vi "DDS_Clock.vi"() -> ()   [LabVIEW 2016] (continued)
"f1 [Hz] CH0"=307800000.0}, {"total time[ms]"=68.04999999999828, "f1 [Hz] CH0"=307800000.0}, {"total time[ms]"=68.09999999999827, "f1 [Hz] CH0"=307599999.99999994}, {"total time[ms]"=68.09999999999827, "f1 [Hz] CH0"=307599999.99999994}, {"total time[ms]"=68.14999999999827, "f1 [Hz] CH0"=307399999.99999994}, {"total time[ms]"=68.14999999999827, "f1 [Hz] CH0"=307399999.99999994}, {"total time[ms]"=68.19999999999827, "f1 [Hz] CH0"=307200000.0}, {"total time[ms]"=68.19999999999827, "f1 [Hz] CH0"=307200000.0}, {"total time[ms]"=68.24999999999827, "f1 [Hz] CH0"=307000000.0}, {"total time[ms]"=68.24999999999827, "f1 [Hz] CH0"=307000000.0}, {"total time[ms]"=68.29999999999826, "f1 [Hz] CH0"=306800000.0}, {"total time[ms]"=68.29999999999826, "f1 [Hz] CH0"=306800000.0}, {"total time[ms]"=68.34999999999826, "f1 [Hz] CH0"=306599999.99999994}, {"total time[ms]"=68.34999999999826, "f1 [Hz] CH0"=306599999.99999994}, {"total time[ms]"=68.39999999999826, "f1 [Hz] CH0"=306400000.0}, {"total time[ms]"=68.39999999999826, "f1 [Hz] CH0"=306400000.0}, {"total time[ms]"=68.44999999999825, "f1 [Hz] CH0"=306200000.0}, {"total time[ms]"=68.44999999999825, "f1 [Hz] CH0"=306200000.0}, {"total time[ms]"=68.49999999999825, "f1 [Hz] CH0"=306000000.0}, {"total time[ms]"=68.49999999999825, "f1 [Hz] CH0"=306000000.0}, {"total time[ms]"=68.54999999999825, "f1 [Hz] CH0"=305800000.0}, {"total time[ms]"=68.54999999999825, "f1 [Hz] CH0"=305800000.0}, {"total time[ms]"=68.59999999999825, "f1 [Hz] CH0"=305599999.99999994}, {"total time[ms]"=68.59999999999825, "f1 [Hz] CH0"=305599999.99999994}, {"total time[ms]"=68.64999999999824, "f1 [Hz] CH0"=305399999.99999994}, {"total time[ms]"=68.64999999999824, "f1 [Hz] CH0"=305399999.99999994}, {"total time[ms]"=68.69999999999824, "f1 [Hz] CH0"=305199999.99999994}, {"total time[ms]"=68.69999999999824, "f1 [Hz] CH0"=305199999.99999994}, {"total time[ms]"=68.74999999999824, "f1 [Hz] CH0"=305000000.0}, {"total time[ms]"=68.74999999999824, "f1 [Hz] CH0"=305000000.0}, {"total time[ms]"=68.79999999999824, "f1 [Hz] CH0"=304800000.0}, {"total time[ms]"=68.79999999999824, "f1 [Hz] CH0"=304800000.0}, {"total time[ms]"=68.84999999999823, "f1 [Hz] CH0"=304599999.99999994}, {"total time[ms]"=68.84999999999823, "f1 [Hz] CH0"=304599999.99999994}, {"total time[ms]"=68.89999999999823, "f1 [Hz] CH0"=304400000.0}, {"total time[ms]"=68.89999999999823, "f1 [Hz] CH0"=304400000.0}, {"total time[ms]"=68.94999999999823, "f1 [Hz] CH0"=304200000.0}, {"total time[ms]"=68.94999999999823, "f1 [Hz] CH0"=304200000.0}, {"total time[ms]"=68.99999999999822, "f1 [Hz] CH0"=304000000.0}, {"total time[ms]"=68.99999999999822, "f1 [Hz] CH0"=304000000.0}, {"total time[ms]"=69.04999999999822, "f1 [Hz] CH0"=303800000.0}, {"total time[ms]"=69.04999999999822, "f1 [Hz] CH0"=303800000.0}, {"total time[ms]"=69.09999999999822, "f1 [Hz] CH0"=303599999.99999994}, {"total time[ms]"=69.09999999999822, "f1 [Hz] CH0"=303599999.99999994}, {"total time[ms]"=69.14999999999822, "f1 [Hz] CH0"=303399999.99999994}, {"total time[ms]"=69.14999999999822, "f1 [Hz] CH0"=303399999.99999994}, {"total time[ms]"=69.19999999999821, "f1 [Hz] CH0"=303199999.99999994}, {"total time[ms]"=69.19999999999821, "f1 [Hz] CH0"=303199999.99999994}, {"total time[ms]"=69.24999999999821, "f1 [Hz] CH0"=303000000.0}, {"total time[ms]"=69.24999999999821, "f1 [Hz] CH0"=303000000.0}, {"total time[ms]"=69.2999999999982, "f1 [Hz] CH0"=302800000.0}, {"total time[ms]"=69.2999999999982, "f1 [Hz] CH0"=302800000.0}, {"total time[ms]"=69.3499999999982, "f1 [Hz] CH0"=302599999.99999994}, {"total time[ms]"=69.3499999999982, "f1 [Hz] CH0"=302599999.99999994}, {"total time[ms]"=69.3999999999982, "f1 [Hz] CH0"=302399999.99999994}, {"total time[ms]"=69.3999999999982, "f1 [Hz] CH0"=302399999.99999994}, {"total time[ms]"=69.4499999999982, "f1 [Hz] CH0"=302200000.0}, {"total time[ms]"=69.4499999999982, "f1 [Hz] CH0"=302200000.0}, {"total time[ms]"=69.4999999999982, "f1 [Hz] CH0"=302000000.0}, {"total time[ms]"=69.4999999999982, "f1 [Hz] CH0"=302000000.0}, {"total time[ms]"=69.54999999999819, "f1 [Hz] CH0"=301800000.0}, {"total time[ms]"=69.54999999999819, "f1 [Hz] CH0"=301800000.0}, {"total time[ms]"=69.59999999999819, "f1 [Hz] CH0"=301599999.99999994}, {"total time[ms]"=69.59999999999819, "f1 [Hz] CH0"=301599999.99999994}, {"total time[ms]"=69.64999999999819, "f1 [Hz] CH0"=301400000.0}, {"total time[ms]"=69.64999999999819, "f1 [Hz] CH0"=301400000.0}, {"total time[ms]"=69.69999999999818, "f1 [Hz] CH0"=301200000.0}, {"total time[ms]"=69.69999999999818, "f1 [Hz] CH0"=301200000.0}, {"total time[ms]"=69.74999999999818, "f1 [Hz] CH0"=301000000.0}, {"total time[ms]"=69.74999999999818, "f1 [Hz] CH0"=301000000.0}, {"total time[ms]"=69.79999999999818, "f1 [Hz] CH0"=300800000.0}, {"total time[ms]"=69.79999999999818, "f1 [Hz] CH0"=300800000.0}, {"total time[ms]"=69.84999999999818, "f1 [Hz] CH0"=300599999.99999994}, {"total time[ms]"=69.84999999999818, "f1 [Hz] CH0"=300599999.99999994}, {"total time[ms]"=69.89999999999817, "f1 [Hz] CH0"=300399999.99999994}, {"total time[ms]"=69.89999999999817, "f1 [Hz] CH0"=300399999.99999994}, {"total time[ms]"=69.94999999999817, "f1 [Hz] CH0"=300199999.99999994}, {"total time[ms]"=69.94999999999817, "f1 [Hz] CH0"=300199999.99999994}, {"total time[ms]"=69.99999999999817, "f1 [Hz] CH0"=300000000.0}, {"total time[ms]"=69.99999999999817, "f1 [Hz] CH0"=300000000.0}, {"total time[ms]"=70.04999999999816, "f1 [Hz] CH0"=300200000.0}, {"total time[ms]"=70.04999999999816, "f1 [Hz] CH0"=300200000.0}, {"total time[ms]"=70.09999999999816, "f1 [Hz] CH0"=300400000.00000006}, {"total time[ms]"=70.09999999999816, "f1 [Hz] CH0"=300400000.00000006}, {"total time[ms]"=70.14999999999816, "f1 [Hz] CH0"=300600000.0}, {"total time[ms]"=70.14999999999816, "f1 [Hz] CH0"=300600000.0}, {"total time[ms]"=70.19999999999816, "f1 [Hz] CH0"=300800000.0}, {"total time[ms]"=70.19999999999816, "f1 [Hz] CH0"=300800000.0}, {"total time[ms]"=70.24999999999815, "f1 [Hz] CH0"=301000000.0}, {"total time[ms]"=70.24999999999815, "f1 [Hz] CH0"=301000000.0}, {"total time[ms]"=70.29999999999815, "f1 [Hz] CH0"=301200000.0}, {"total time[ms]"=70.29999999999815, "f1 [Hz] CH0"=301200000.0}, {"total time[ms]"=70.34999999999815, "f1 [Hz] CH0"=301400000.00000006}, {"total time[ms]"=70.34999999999815, "f1 [Hz] CH0"=301400000.00000006}, {"total time[ms]"=70.39999999999814, "f1 [Hz] CH0"=301600000.00000006}, {"total time[ms]"=70.39999999999814, "f1 [Hz] CH0"=301600000.00000006}, {"total time[ms]"=70.44999999999814, "f1 [Hz] CH0"=301800000.00000006}, {"total time[ms]"=70.44999999999814, "f1 [Hz] CH0"=301800000.00000006}, {"total time[ms]"=70.49999999999814, "f1 [Hz] CH0"=302000000.0}, {"total time[ms]"=70.49999999999814, "f1 [Hz] CH0"=302000000.0}, {"total time[ms]"=70.54999999999814, "f1 [Hz] CH0"=302200000.0}, {"total time[ms]"=70.54999999999814, "f1 [Hz] CH0"=302200000.0}, {"total time[ms]"=70.59999999999813, "f1 [Hz] CH0"=302400000.00000006}, {"total time[ms]"=70.59999999999813, "f1 [Hz] CH0"=302400000.00000006}, {"total time[ms]"=70.64999999999813, "f1 [Hz] CH0"=302600000.00000006}, {"total time[ms]"=70.64999999999813, "f1 [Hz] CH0"=302600000.00000006}, {"total time[ms]"=70.69999999999813, "f1 [Hz] CH0"=302800000.0}, {"total time[ms]"=70.69999999999813, "f1 [Hz] CH0"=302800000.0}, {"total time[ms]"=70.74999999999812, "f1 [Hz] CH0"=303000000.0}, {"total time[ms]"=70.74999999999812, "f1 [Hz] CH0"=303000000.0}, {"total time[ms]"=70.79999999999812, "f1 [Hz] CH0"=303200000.0}, {"total time[ms]"=70.79999999999812, "f1 [Hz] CH0"=303200000.0}, {"total time[ms]"=70.84999999999812, "f1 [Hz] CH0"=303400000.00000006}, {"total time[ms]"=70.84999999999812, "f1 [Hz] CH0"=303400000.00000006}, {"total time[ms]"=70.89999999999812, "f1 [Hz] CH0"=303600000.0}, {"total time[ms]"=70.89999999999812, "f1 [Hz] CH0"=303600000.0}, {"total time[ms]"=70.94999999999811, "f1 [Hz] CH0"=303800000.0}, {"total time[ms]"=70.94999999999811, "f1 [Hz] CH0"=303800000.0}, {"total time[ms]"=70.99999999999811, "f1 [Hz] CH0"=304000000.0}, {"total time[ms]"=70.99999999999811, "f1 [Hz] CH0"=304000000.0}, {"total time[ms]"=71.04999999999811, "f1 [Hz] CH0"=304200000.0}, {"total time[ms]"=71.04999999999811, "f1 [Hz] CH0"=304200000.0}, {"total time[ms]"=71.0999999999981, "f1 [Hz] CH0"=304400000.00000006}, {"total time[ms]"=71.0999999999981, "f1 [Hz] CH0"=304400000.00000006}, {"total time[ms]"=71.1499999999981, "f1 [Hz] CH0"=304600000.00000006}, {"total time[ms]"=71.1499999999981, "f1 [Hz] CH0"=304600000.00000006}, {"total time[ms]"=71.1999999999981, "f1 [Hz] CH0"=304800000.00000006}, {"total time[ms]"=71.1999999999981, "f1 [Hz] CH0"=304800000.00000006}, {"total time[ms]"=71.2499999999981, "f1 [Hz] CH0"=305000000.0}, {"total time[ms]"=71.2499999999981, "f1 [Hz] CH0"=305000000.0}, {"total time[ms]"=71.2999999999981, "f1 [Hz] CH0"=305200000.0}, {"total time[ms]"=71.2999999999981, "f1 [Hz] CH0"=305200000.0}, {"total time[ms]"=71.34999999999809, "f1 [Hz] CH0"=305400000.00000006}, {"total time[ms]"=71.34999999999809, "f1 [Hz] CH0"=305400000.00000006}, {"total time[ms]"=71.39999999999809, "f1 [Hz] CH0"=305600000.0}, {"total time[ms]"=71.39999999999809, "f1 [Hz] CH0"=305600000.0}, {"total time[ms]"=71.44999999999808, "f1 [Hz] CH0"=305800000.0}, {"total time[ms]"=71.44999999999808, "f1 [Hz] CH0"=305800000.0}, {"total time[ms]"=71.49999999999808, "f1 [Hz] CH0"=306000000.0}, {"total time[ms]"=71.49999999999808, "f1 [Hz] CH0"=306000000.0}, {"total time[ms]"=71.54999999999808, "f1 [Hz] CH0"=306200000.0}, {"total time[ms]"=71.54999999999808, "f1 [Hz] CH0"=306200000.0}, {"total time[ms]"=71.59999999999808, "f1 [Hz] CH0"=306400000.00000006}, {"total time[ms]"=71.59999999999808, "f1 [Hz] CH0"=306400000.00000006}, {"total time[ms]"=71.64999999999807, "f1 [Hz] CH0"=306600000.00000006}, {"total time[ms]"=71.64999999999807, "f1 [Hz] CH0"=306600000.00000006}, {"total time[ms]"=71.69999999999807, "f1 [Hz] CH0"=306800000.00000006}, {"total time[ms]"=71.69999999999807, "f1 [Hz] CH0"=306800000.00000006}, {"total time[ms]"=71.74999999999807, "f1 [Hz] CH0"=307000000.0}, {"total time[ms]"=71.74999999999807, "f1 [Hz] CH0"=307000000.0}, {"total time[ms]"=71.79999999999806, "f1 [Hz] CH0"=307200000.0}, {"total time[ms]"=71.79999999999806, "f1 [Hz] CH0"=307200000.0}, {"total time[ms]"=71.84999999999806, "f1 [Hz] CH0"=307400000.00000006}, {"total time[ms]"=71.84999999999806, "f1 [Hz] CH0"=307400000.00000006}, {"total time[ms]"=71.89999999999806, "f1 [Hz] CH0"=307600000.00000006}, {"total time[ms]"=71.89999999999806, "f1 [Hz] CH0"=307600000.00000006}, {"total time[ms]"=71.94999999999806, "f1 [Hz] CH0"=307800000.0}, {"total time[ms]"=71.94999999999806, "f1 [Hz] CH0"=307800000.0}, {"total time[ms]"=71.99999999999805, "f1 [Hz] CH0"=308000000.0}, {"total time[ms]"=71.99999999999805, "f1 [Hz] CH0"=308000000.0}, {"total time[ms]"=72.04999999999805, "f1 [Hz] CH0"=308200000.0}, {"total time[ms]"=72.04999999999805, "f1 [Hz] CH0"=308200000.0}, {"total time[ms]"=72.09999999999805, "f1 [Hz] CH0"=308400000.00000006}, {"total time[ms]"=72.09999999999805, "f1 [Hz] CH0"=308400000.00000006}, {"total time[ms]"=72.14999999999804, "f1 [Hz] CH0"=308600000.0}, {"total time[ms]"=72.14999999999804, "f1 [Hz] CH0"=308600000.0}, {"total time[ms]"=72.19999999999804, "f1 [Hz] CH0"=308800000.0}, {"total time[ms]"=72.19999999999804, "f1 [Hz] CH0"=308800000.0}, {"total time[ms]"=72.24999999999804, "f1 [Hz] CH0"=309000000.0}, {"total time[ms]"=72.24999999999804, "f1 [Hz] CH0"=309000000.0}, {"total time[ms]"=72.29999999999804, "f1 [Hz] CH0"=309200000.0}, {"total time[ms]"=72.29999999999804, "f1 [Hz] CH0"=309200000.0}, {"total time[ms]"=72.34999999999803, "f1 [Hz] CH0"=309400000.00000006}, {"total time[ms]"=72.34999999999803, "f1 [Hz] CH0"=309400000.00000006}, {"total time[ms]"=72.39999999999803, "f1 [Hz] CH0"=309600000.00000006}, {"total time[ms]"=72.39999999999803, "f1 [Hz] CH0"=309600000.00000006}, {"total time[ms]"=72.44999999999803, "f1 [Hz] CH0"=309800000.00000006}, {"total time[ms]"=72.44999999999803, "f1 [Hz] CH0"=309800000.00000006}, {"total time[ms]"=72.49999999999802, "f1 [Hz] CH0"=310000000.0}, {"total time[ms]"=72.49999999999802, "f1 [Hz] CH0"=310000000.0}, {"total time[ms]"=72.54999999999802, "f1 [Hz] CH0"=310200000.0}, {"total time[ms]"=72.54999999999802, "f1 [Hz] CH0"=310200000.0}, {"total time[ms]"=72.59999999999802, "f1 [Hz] CH0"=310400000.00000006}, {"total time[ms]"=72.59999999999802, "f1 [Hz] CH0"=310400000.00000006}, {"total time[ms]"=72.64999999999802, "f1 [Hz] CH0"=310600000.0}, {"total time[ms]"=72.64999999999802, "f1 [Hz] CH0"=310600000.0}, {"total time[ms]"=72.69999999999801, "f1 [Hz] CH0"=310800000.0}, {"total time[ms]"=72.69999999999801, "f1 [Hz] CH0"=310800000.0}, {"total time[ms]"=72.74999999999801, "f1 [Hz] CH0"=311000000.0}, {"total time[ms]"=72.74999999999801, "f1 [Hz] CH0"=311000000.0}, {"total time[ms]"=72.79999999999801, "f1 [Hz] CH0"=311200000.0}, {"total time[ms]"=72.79999999999801, "f1 [Hz] CH0"=311200000.0}, {"total time[ms]"=72.849999999998, "f1 [Hz] CH0"=311400000.00000006}, {"total time[ms]"=72.849999999998, "f1 [Hz] CH0"=311400000.00000006}, {"total time[ms]"=72.899999999998, "f1 [Hz] CH0"=311600000.00000006}, {"total time[ms]"=72.899999999998, "f1 [Hz] CH0"=311600000.00000006}, {"total time[ms]"=72.949999999998, "f1 [Hz] CH0"=311800000.00000006}, {"total time[ms]"=72.949999999998, "f1 [Hz] CH0"=311800000.00000006}, {"total time[ms]"=72.999999999998, "f1 [Hz] CH0"=312000000.0}, {"total time[ms]"=72.999999999998, "f1 [Hz] CH0"=312000000.0}, {"total time[ms]"=73.049999999998, "f1 [Hz] CH0"=312200000.0}, {"total time[ms]"=73.049999999998, "f1 [Hz] CH0"=312200000.0}, {"total time[ms]"=73.09999999999799, "f1 [Hz] CH0"=312400000.00000006}, {"total time[ms]"=73.09999999999799, "f1 [Hz] CH0"=312400000.00000006}, {"total time[ms]"=73.14999999999799, "f1 [Hz] CH0"=312600000.00000006}, {"total time[ms]"=73.14999999999799, "f1 [Hz] CH0"=312600000.00000006}, {"total time[ms]"=73.19999999999798, "f1 [Hz] CH0"=312800000.0}, {"total time[ms]"=73.19999999999798, "f1 [Hz] CH0"=312800000.0}, {"total time[ms]"=73.24999999999798, "f1 [Hz] CH0"=313000000.0}, {"total time[ms]"=73.24999999999798, "f1 [Hz] CH0"=313000000.0}, {"total time[ms]"=73.29999999999798, "f1 [Hz] CH0"=313200000.0}, {"total time[ms]"=73.29999999999798, "f1 [Hz] CH0"=313200000.0}, {"total time[ms]"=73.34999999999798, "f1 [Hz] CH0"=313400000.00000006}, {"total time[ms]"=73.34999999999798, "f1 [Hz] CH0"=313400000.00000006}, {"total time[ms]"=73.39999999999797, "f1 [Hz] CH0"=313600000.0}, {"total time[ms]"=73.39999999999797, "f1 [Hz] CH0"=313600000.0}, {"total time[ms]"=73.44999999999797, "f1 [Hz] CH0"=313800000.0}, {"total time[ms]"=73.44999999999797, "f1 [Hz] CH0"=313800000.0}, {"total time[ms]"=73.49999999999797, "f1 [Hz] CH0"=314000000.0}, {"total time[ms]"=73.49999999999797, "f1 [Hz] CH0"=314000000.0}, {"total time[ms]"=73.54999999999797, "f1 [Hz] CH0"=314200000.0}, {"total time[ms]"=73.54999999999797, "f1 [Hz] CH0"=314200000.0}, {"total time[ms]"=73.59999999999796, "f1 [Hz] CH0"=314400000.00000006}, {"total time[ms]"=73.59999999999796, "f1 [Hz] CH0"=314400000.00000006}, {"total time[ms]"=73.64999999999796, "f1 [Hz] CH0"=314600000.00000006}, {"total time[ms]"=73.64999999999796, "f1 [Hz] CH0"=314600000.00000006}, {"total time[ms]"=73.69999999999796, "f1 [Hz] CH0"=314800000.00000006}, {"total time[ms]"=73.69999999999796, "f1 [Hz] CH0"=314800000.00000006}, {"total time[ms]"=73.74999999999795, "f1 [Hz] CH0"=315000000.0}, {"total time[ms]"=73.74999999999795, "f1 [Hz] CH0"=315000000.0}, {"total time[ms]"=73.79999999999795, "f1 [Hz] CH0"=315200000.0}, {"total time[ms]"=73.79999999999795, "f1 [Hz] CH0"=315200000.0}, {"total time[ms]"=73.84999999999795, "f1 [Hz] CH0"=315400000.00000006}, {"total time[ms]"=73.84999999999795, "f1 [Hz] CH0"=315400000.00000006}, {"total time[ms]"=73.89999999999795, "f1 [Hz] CH0"=315600000.0}, {"total time[ms]"=73.89999999999795, "f1 [Hz] CH0"=315600000.0}, {"total time[ms]"=73.94999999999794, "f1 [Hz] CH0"=315800000.0}, {"total time[ms]"=73.94999999999794, "f1 [Hz] CH0"=315800000.0}, {"total time[ms]"=73.99999999999794, "f1 [Hz] CH0"=316000000.0}, {"total time[ms]"=73.99999999999794, "f1 [Hz] CH0"=316000000.0}, {"total time[ms]"=74.04999999999794, "f1 [Hz] CH0"=316200000.0}, {"total time[ms]"=74.04999999999794, "f1 [Hz] CH0"=316200000.0}, {"total time[ms]"=74.09999999999793, "f1 [Hz] CH0"=316400000.00000006}, {"total time[ms]"=74.09999999999793, "f1 [Hz] CH0"=316400000.00000006}, {"total time[ms]"=74.14999999999793, "f1 [Hz] CH0"=316600000.00000006}, {"total time[ms]"=74.14999999999793, "f1 [Hz] CH0"=316600000.00000006}, {"total time[ms]"=74.19999999999793, "f1 [Hz] CH0"=316800000.00000006}, {"total time[ms]"=74.19999999999793, "f1 [Hz] CH0"=316800000.00000006}, {"total time[ms]"=74.24999999999793, "f1 [Hz] CH0"=317000000.0}, {"total time[ms]"=74.24999999999793, "f1 [Hz] CH0"=317000000.0}, {"total time[ms]"=74.29999999999792, "f1 [Hz] CH0"=317200000.0}, {"total time[ms]"=74.29999999999792, "f1 [Hz] CH0"=317200000.0}, {"total time[ms]"=74.34999999999792, "f1 [Hz] CH0"=317400000.00000006}, {"total time[ms]"=74.34999999999792, "f1 [Hz] CH0"=317400000.00000006}, {"total time[ms]"=74.39999999999792, "f1 [Hz] CH0"=317600000.00000006}, {"total time[ms]"=74.39999999999792, "f1 [Hz] CH0"=317600000.00000006}, {"total time[ms]"=74.44999999999791, "f1 [Hz] CH0"=317800000.0}, {"total time[ms]"=74.44999999999791, "f1 [Hz] CH0"=317800000.0}, {"total time[ms]"=74.49999999999791, "f1 [Hz] CH0"=318000000.0}, {"total time[ms]"=74.49999999999791, "f1 [Hz] CH0"=318000000.0}, {"total time[ms]"=74.54999999999791, "f1 [Hz] CH0"=318200000.0}, {"total time[ms]"=74.54999999999791, "f1 [Hz] CH0"=318200000.0}, {"total time[ms]"=74.5999999999979, "f1 [Hz] CH0"=318400000.00000006}, {"total time[ms]"=74.5999999999979, "f1 [Hz] CH0"=318400000.00000006}, {"total time[ms]"=74.6499999999979, "f1 [Hz] CH0"=318600000.0}, {"total time[ms]"=74.6499999999979, "f1 [Hz] CH0"=318600000.0}, {"total time[ms]"=74.6999999999979, "f1 [Hz] CH0"=318800000.0}, {"total time[ms]"=74.6999999999979, "f1 [Hz] CH0"=318800000.0}, {"total time[ms]"=74.7499999999979, "f1 [Hz] CH0"=319000000.0}, {"total time[ms]"=74.7499999999979, "f1 [Hz] CH0"=319000000.0}, {"total time[ms]"=74.7999999999979, "f1 [Hz] CH0"=319200000.0}, {"total time[ms]"=74.7999999999979, "f1 [Hz] CH0"=319200000.0}, {"total time[ms]"=74.84999999999789, "f1 [Hz] CH0"=319400000.00000006}, {"total time[ms]"=74.84999999999789, "f1 [Hz] CH0"=319400000.00000006}, {"total time[ms]"=74.89999999999789, "f1 [Hz] CH0"=319600000.00000006}, {"total time[ms]"=74.89999999999789, "f1 [Hz] CH0"=319600000.00000006}, {"total time[ms]"=74.94999999999789, "f1 [Hz] CH0"=319800000.00000006}, {"total time[ms]"=74.94999999999789, "f1 [Hz] CH0"=319800000.00000006}, {"total time[ms]"=74.99999999999788, "f1 [Hz] CH0"=320000000.0}, {"total time[ms]"=74.99999999999788, "f1 [Hz] CH0"=320000000.0}, {"total time[ms]"=75.04999999999788, "f1 [Hz] CH0"=319800000.0}, {"total time[ms]"=75.04999999999788, "f1 [Hz] CH0"=319800000.0}, {"total time[ms]"=75.09999999999788, "f1 [Hz] CH0"=319599999.99999994}, {"total time[ms]"=75.09999999999788, "f1 [Hz] CH0"=319599999.99999994}, {"total time[ms]"=75.14999999999787, "f1 [Hz] CH0"=319400000.0}, {"total time[ms]"=75.14999999999787, "f1 [Hz] CH0"=319400000.0}, {"total time[ms]"=75.19999999999787, "f1 [Hz] CH0"=319200000.0}, {"total time[ms]"=75.19999999999787, "f1 [Hz] CH0"=319200000.0}, {"total time[ms]"=75.24999999999787, "f1 [Hz] CH0"=319000000.0}, {"total time[ms]"=75.24999999999787, "f1 [Hz] CH0"=319000000.0}, {"total time[ms]"=75.29999999999787, "f1 [Hz] CH0"=318800000.0}, {"total time[ms]"=75.29999999999787, "f1 [Hz] CH0"=318800000.0}, {"total time[ms]"=75.34999999999786, "f1 [Hz] CH0"=318599999.99999994}, {"total time[ms]"=75.34999999999786, "f1 [Hz] CH0"=318599999.99999994}, {"total time[ms]"=75.39999999999786, "f1 [Hz] CH0"=318399999.99999994}, {"total time[ms]"=75.39999999999786, "f1 [Hz] CH0"=318399999.99999994}, {"total time[ms]"=75.44999999999786, 
